vi "PSTR-Show Gain Curves.vi"(0 "Data":T1, 5 "XYGraph":refnum<vi>, 7 "Freq":u16) -> ()   [LabVIEW 2020]
uses:
  Typedefs/PSTR-Data.ctl
  Typedefs/PSTR-Model Fit.ctl
  Typedefs/PSTR-Fit Parameters.ctl
panel:
  # "NF x NL x 2 x Npts"
  # "NF x NL x Npts"
  # "NF x NL"
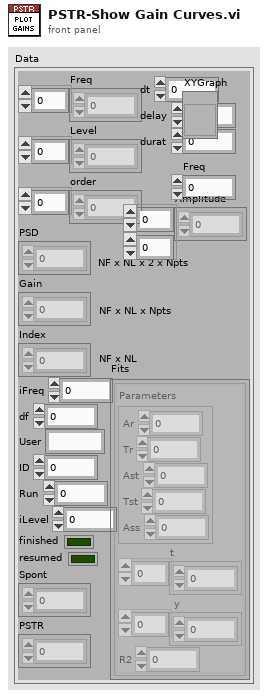
[diagram p1: front panel]
types:
  T1 = typedef "PSTR-Data.ctl" = cluster{"Freq":dbl[], "Level":dbl[], "order":i32[], "PSD":dbl[][][][], "Gain":dbl[][][], "Index":dbl[][], "iFreq":i32, "df":dbl, "User":string, "ID":i32, "Run":i32, "iLevel":i32, "finished":bool, "resumed":bool, "Spont":dbl[][], "PSTR":dbl[][][], "dt":dbl, "delay":dbl, "durat":dbl, "Fits":T2[][], "Amplitude":dbl[][]}
  T2 = typedef "PSTR-Model Fit.ctl" = cluster{"Parameters":T3, "t":dbl[], "y":dbl[], "R2":dbl}
  T3 = typedef "PSTR-Fit Parameters.ctl" = cluster{"Ar":dbl, "Tr":dbl, "Ast":dbl, "Tst":dbl, "Ass":dbl}
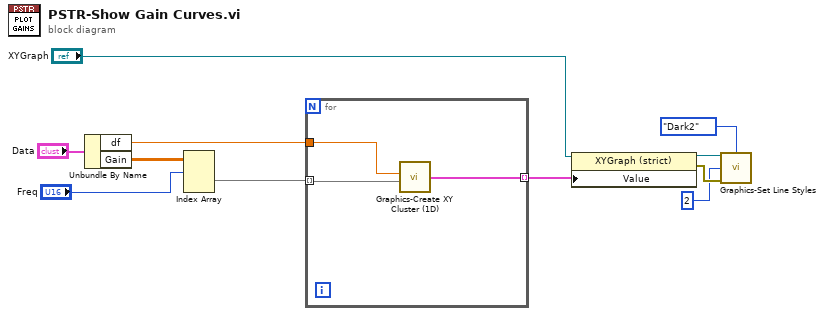
[diagram p0: block diagram]
diagram:
  n1 = Unbundle By Name("Data") -> ("df"=w7:dbl, "Gain"=w10:dbl[][][])
  n2 = Index Array(array=w10, index (dim 0)="Freq") -> (element=w8:dbl[][])  [unwired: 2 in]
  n3 = for {
    tunnel: w8 -> [w13] mode=indexing
    tunnel: w7 -> [w14]
    tunnel: [w12] -> w6 mode=indexing
    n4 = call "Graphics-Create XY Cluster (1D).vi"("Array"=w13, "dx"=w14) -> ("XY cluster"=w12:cluster{"Array":dbl[], "Array":dbl[]})  [unwired: 2 in]
  }
  n5 = property class="XYGraph (strict)"(reference="XYGraph", "Value"=w6) -> (reference out=w3:refnum<vi>, error out=w4:errorcluster)  [unwired: 1 in]
  n6 = call "Graphics-Set Line Styles.vi"("XY Graph"=w3, "Map"=enum16{"User", "Prism", "Kelly", "Dark2"}."Dark2", "Plot.Line Width"=u8 2, "error in (no error)"=w4) -> ()  [unwired: 10 in, 2 out]
